vi "Piston for cans.vi"(8 "error in (no error)":errorcluster, 10 "Button 5":bool, 11 "Button 4":bool) -> (0 "error out":errorcluster)   [LabVIEW 2014]
uses:
  <vilib>/Rock Robotics/WPI/Solenoid/Deprecated/WPI_SolenoidGetBool.vi
  <vilib>/Rock Robotics/WPI/Solenoid/Deprecated/WPI_SolenoidSetBool.vi
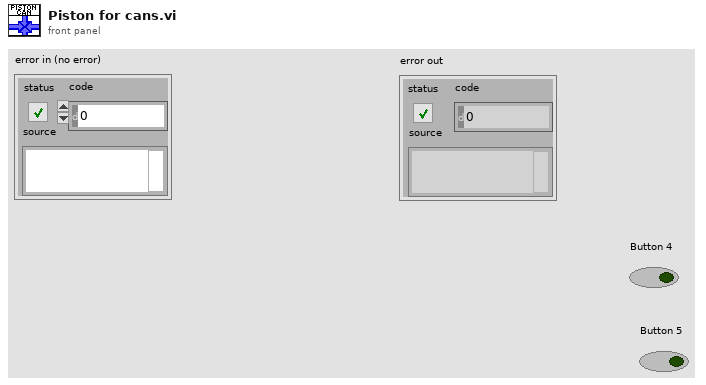
[diagram p1: front panel]
types:
  T1 = typedef "WPI_SolenoidDevRef.ctl" = cluster{"DevStatus":errorcluster, "Pneumatics Control Module":u8, "Forward Solenoid Channel":T2, "Reverse Solenoid Channel":T2}
  T2 = typedef "WPI_SolenoidChannel.ctl" = enum8{"Solenoid 0", "Solenoid 1", "Solenoid 2", "Solenoid 3", "Solenoid 4", "Solenoid 5", "Solenoid 6", "Solenoid 7", "Invalid"}
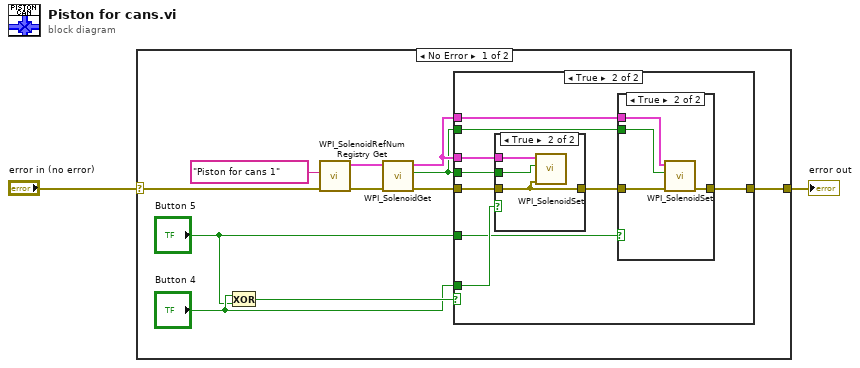
[diagram p0: block diagram]
diagram:
  n1 = case shown="No Error" "error in (no error)" {
    selector: "error in (no error)" -> [w12 w33]
    tunnel: [w3 w33] -> w1
    frame No Error {
      n2 = Exclusive Or(1:"Button 5", 2:"Button 4") -> (0:w9:bool)
      n3 = call <vilib>:"WPI_SolenoidRefNum Registry Get.vi"("error in (no error)"=w12, "refnum name"="Piston for cans 1") -> ("error out"=w10:errorcluster, "SolenoidDevRef"=w11:T1)  [unwired: 8 in]
      n4 = call-poly <vilib>:"WPI_SolenoidGet.vi"("error in (no error)"=w10, "SolenoidDevRef"=w11) -> ("error out"=w6:errorcluster, "Value"=w4:bool, "SolenoidDevRef"=w5:T1)  [unwired: 7 in]
      n5 = case shown="True" w9 {
        tunnel: "Button 4" -> [_ w23]
        tunnel: "Button 5" -> [_ w22]
        tunnel: w4 -> [_ w21]
        tunnel: w5 -> [_ w20]
        tunnel: w6 -> [w14 w19]
        tunnel: w5 -> [_ w18]
        tunnel: w4 -> [_ w17]
        tunnel: [w14 w15] -> w3
        frame False {
        }
        frame True {
          n6 = case shown="True" w23 {
            tunnel: w21 -> [_ w32]
            tunnel: w20 -> [_ w31]
            tunnel: w19 -> [w29 w30]
            tunnel: [w29 w30] -> w16
            frame False {
            }
            frame True {
              n7 = call-poly <vilib>:"WPI_SolenoidSet.vi"("error in (no error)"=w30, "Value"=w32, "SolenoidDevRef"=w31) -> ()  [unwired: 7 in, 2 out]
            }
          }
          n8 = case shown="True" w22 {
            tunnel: w18 -> [_ w28]
            tunnel: w17 -> [_ w27]
            tunnel: w16 -> [w24 w26]
            tunnel: [w24 w25] -> w15
            frame False {
            }
            frame True {
              n9 = call-poly <vilib>:"WPI_SolenoidSet.vi"("error in (no error)"=w26, "Value"=w27, "SolenoidDevRef"=w28) -> ("error out"=w25:errorcluster)  [unwired: 7 in, 1 out]
            }
          }
        }
      }
    }
    frame Error {
      # "This is what to do if there is an error.  Usually it is nothing."
    }
  }
  "error out" <- w1
